vi "SLSC_Device_Mismatch_Error_Message.vi"(9 "Name":string, 10 "Slot Number":string, 11 "Product Name":string) -> (3 "String":string)   [LabVIEW 2020, in "SLSC-12201 DIO Engine.lvlib"]
uses:
  SLSC-12201 DIO Engine.lvlib
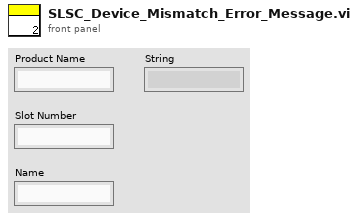
[diagram p1: front panel]
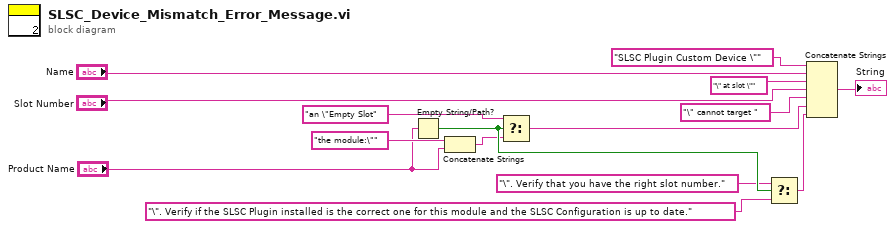
[diagram p0: block diagram]
diagram:
  n1 = Empty String/Path?(string/path="Product Name") -> (empty?=w12:bool)
  n2 = Concatenate Strings("the module:\"" ("error message (\"\")"), "Product Name") -> (w6:string)
  n3 = Select(t="an \"Empty Slot" ("error message (\"\")"), s=w12, f=w6) -> (s? t:f=w5:string)
  n4 = Select(t="\". Verify that you have the right slot number." ("string"), s=w12, f="\". Verify if the SLSC Plugin installed is the correct one for this module and the SLSC Configuration is up to date." ("string")) -> (s? t:f=w11:string)
  n5 = Concatenate Strings("SLSC Plugin Custom Device \"" ("error message (\"\")"), "Name", "\" at slot \"" ("error message (\"\")"), "Slot Number", "\" cannot target " ("error message (\"\")"), w5, w11) -> (→"String":string)
